vi "TCP_receive.vi"(8 "error in (no error)":errorcluster, 10 "queue":refnum<queue>) -> (0 "error out":errorcluster)   [LabVIEW 2013, in "Experiment.lvclass"]
uses:
  Experiment.lvclass
  Globals.vi
  TCP_IP/TCP_IP.lvclass
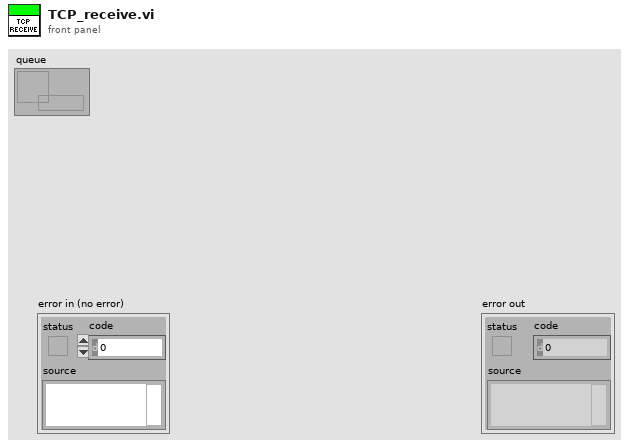
[diagram p1: front panel]
types:
  T1 = enum16{"Clear and Continue", "Clear and Restart", "Clear and Stop", "Halt"}
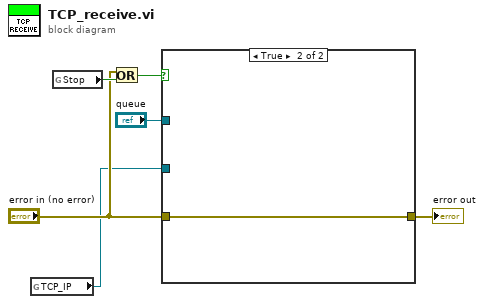
[diagram p0: block diagram]
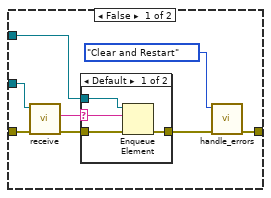
[diagram p2: hidden frame]
diagram:
  n1 = global read "Globals.vi" "TCP_IP"() -> (w1:refnum<class "TCP_IP.lvclass">)
  n2 = global read "Globals.vi" "Stop"() -> (w3:bool)
  n3 = Or(x="error in (no error)", y=w3) -> (x .or. y?=w4:bool)
  n4 = case shown="True" w4 {
    tunnel: [w14 w20] -> w6
    tunnel: w1 -> [w8 _]
    tunnel: "queue" -> [w13 _]
    tunnel: "error in (no error)" -> [w9 w20]
    frame False {
      n5 = call "receive.vi"("error in (no error)"=w9, "TCP_IP.lvclass"=w8) -> ("error out"=w11:errorcluster, "data out"=w12:string)  [unwired: 8 in]
      n6 = case shown="Default" w12 {
        selector: w12 -> [w15 _]
        tunnel: w13 -> [w18 _]
        tunnel: w11 -> [w17 w19]
        tunnel: [w16 w19] -> w10
        frame Default {
          n7 = Enqueue Element(queue=w18, element=w15, error in (no error)=w17) -> (error out=w16:errorcluster)  [unwired: 1 in, 2 out]
        }
        frame "" {
        }
      }
      n8 = call "handle_errors.vi"("error in (no error)"=w10, "Action?"=T1."Clear and Restart") -> ("error out"=w14:errorcluster)  [unwired: 9 in]
    }
    frame True {
    }
  }
  "error out" <- w6
